vi "Optoelectronic.vi"(0 "Function":T30=enum."Set Parameter Analyzer", 5 "Light Settings":T7={"Laser Settings"={"Wavelength"=enum."365 nm", "Power"=enum."100%"}, "Spectrometer Settings"={"Confocal Hole Size (µm)"=150.0, "Grating"=1, "Detector"=enum."InGaAs Array"}} {"Spectrometer Settings"."Grating" items=["1800 l/mm", "150 l/mm"]}, 7 "Electrical Settings":T14={"SMU1 - Sampling"={"Source"=10.0, "Compliance"=1e-05, "Mode"=0, "Function"=FALSE}, "SMU2 - Sampling"={"Source"=10.0, "Compliance"=1e-05, "Mode"=0, "Function"=FALSE}, "SMU3 - Sampling"={"Source"=10.0, "Compliance"=1e-05, "Mode"=0, "Function"=FALSE}, "SMU4 - Sampling"={"Source"=10.0, "Compliance"=1e-05, "Mode"=0, "Function"=FALSE}} {"SMU4 - Sampling"."Mode" items=["V", "I", "Common"]; "SMU4 - Sampling"."Compliance" format="%^.2e"; "SMU4 - Sampling"."Source" format="%^.3e"; "SMU3 - Sampling"."Mode" items=["V", "I", "Common"]; "SMU3 - Sampling"."Compliance" format="%^.2e"; "SMU3 - Sampling"."Source" format="%^.3e"; "SMU2 - Sampling"."Mode" items=["V", "I", "Common"]; "SMU2 - Sampling"."Compliance" format="%^.2e"; "SMU2 - Sampling"."Source" format="%^.3e"; "SMU1 - Sampling"."Mode" items=["V", "I", "Common"]; "SMU1 - Sampling"."Compliance" format="%^.2e"; "SMU1 - Sampling"."Source" format="%^.3e"}, 9 "Acquisition Settings":T32={"Acquisition Mode"=enum."Single Window", "Spectal Position (nm)"=480.0, "From (nm)"=632.0, "To (nm)"=1000.0, "Integration Time (s)"=3.0, "Number of Accumulations"=3, "AutoScanning"=FALSE, "Spike Removal"=FALSE}, 11 "error in (no error)":errorcluster, 12 "Message Queues":T16, 13 "Notifiers":T17, 14 "Refnums":T1) -> (15 "error out":errorcluster)   [LabVIEW 2014]
uses:
  Hardware Control/Spectrometer/Acquisition Settings.ctl
  Hardware Control/Parameter Analyzer/Parameter Analyzer Sampling Parameters.ctl
  Optoelectronic Funtions.ctl
  support/Notifiers/Notifiers.ctl
  support/Message Handler Loop Notifiers.ctl
  Hardware Control/Parameter Analyzer/Parameter Analyzer Notifiers.ctl
  Hardware Control/Switching Matrix/Switching Matrix Notifiers.ctl
  Hardware Control/Stress Control/StressControl Notifiers.ctl
  Hardware Control/Spectrometer/Spectrometer Notifiers.ctl
  Hardware Control/Switches and Mirrors/SwitchesMirrors Notifiers.ctl
  Hardware Control/Camera/Camera Notifiers.ctl
  Hardware Control/XYZ Stage/XYZ Notifications.ctl
  Hardware Control/Autofocus/Autofocus Notifiers.ctl
  Optoelectronic Notifiers.ctl
  Save Data/SaveData Notifiers.ctl
  Instrument Sequence/Instrument Sequence Notifiers.ctl
  support/Message Queue/All Message Queues.ctl
  support/Message Queue/Message Cluster.ctl
  Optoelectronic Electrical Settings.ctl
  Hardware Control/Parameter Analyzer/Parameter Analyzer SMU Sampling.ctl
  Optoelectronic Light Settings.ctl
  Optoelectronic Laser Settings.ctl
  Hardware Control/Spectrometer/Laser.ctl
  Optoelectronic Power.ctl
  Hardware Control/Spectrometer/Grating Detector Settings.ctl
  Hardware Control/Spectrometer/Grating.ctl
  Hardware Control/Spectrometer/Detector.ctl
  Hardware Control/Parameter Analyzer/Voltage Plot.ctl
  Hardware Control/Parameter Analyzer/Current Plot.ctl
  support/Instrument Status.ctl
  Optoelectronic Refnums.ctl
  Plot Data/Optical Spectrum Plot Refnum.ctl
  Plot Data/Electrical Data Plot Refnums.ctl
  support/Status of All Instruments.ctl
  Hardware Control/Parameter Analyzer/Parameter Analyzer Data.ctl
  Hardware Control/Parameter Analyzer/Parameter Analyzer Config.ctl
  Hardware Control/Parameter Analyzer/Parameter Analyzer Integration Parameters.ctl
  Hardware Control/Parameter Analyzer/Parameter Analyzer SMU Sweeping.ctl
  Hardware Control/Parameter Analyzer/Parameter Analyzer Sweep Spacing.ctl
  Hardware Control/Parameter Analyzer/Parameter Analyzer SMU Range.ctl
  Hardware Control/Parameter Analyzer/Parameter Analyzer Stop Sampling Conditions.ctl
  Hardware Control/Parameter Analyzer/Parameter Analyzer Refnums.ctl
  Hardware Control/Parameter Analyzer/Parameter Analyzer Initialization.ctl
  Hardware Control/Switching Matrix/Switching Matrix Data.ctl
  Hardware Control/Switching Matrix/Switching Matrix Config.ctl
  Hardware Control/Switching Matrix/Switching Matrix Refnums.ctl
  Hardware Control/Switching Matrix/Switching Matrix Initialization.ctl
  Hardware Control/Stress Control/StressControl Data.ctl
  Hardware Control/Stress Control/StressControl Config.ctl
  Hardware Control/Stress Control/StressControl Refnums.ctl
  Hardware Control/Stress Control/StressControl Initialization.ctl
  Hardware Control/Spectrometer/Spectrometer Data.ctl
  Hardware Control/Spectrometer/Spectrometer Config.ctl
  Hardware Control/Spectrometer/Laser Settings.ctl
  Hardware Control/Spectrometer/Filter.ctl
  Hardware Control/Spectrometer/Spectrometer Refnum.ctl
  Hardware Control/Spectrometer/Spectrometer Initialization.ctl
  Hardware Control/Switches and Mirrors/SwitchesMirrors Data.ctl
  Hardware Control/Switches and Mirrors/SwitchesMirrors Config.ctl
  Hardware Control/Switches and Mirrors/SwitchesMirrors Status.ctl
  Hardware Control/Switches and Mirrors/SwitchesMirrors Refnum.ctl
  Hardware Control/Switches and Mirrors/SwitchesMirrors Initialize.ctl
  Hardware Control/Camera/Camera Data.ctl
  Hardware Control/Camera/Camera Config.ctl
  Hardware Control/Camera/Camera Settings.ctl
  Hardware Control/Camera/Camera Refnums.ctl
  Hardware Control/Camera/Camera Initialization.ctl
  Hardware Control/XYZ Stage/XYZ Data.ctl
  Hardware Control/XYZ Stage/XYZ Config.ctl
  Hardware Control/XYZ Stage/XYZ Connection Settings.ctl
  Hardware Control/XYZ Stage/XYZ Stage Control.ctl
  Hardware Control/XYZ Stage/XYZ Coordinate Control.ctl
  Hardware Control/XYZ Stage/XYZ Refnums.ctl
  Hardware Control/XYZ Stage/XYZ Initialization.ctl
  Hardware Control/Autofocus/AutoFocus Data.ctl
  Hardware Control/Autofocus/AutoFocus Config.ctl
  Hardware Control/Autofocus/ZScan.ctl
  <vilib>/Analysis/Matrix/Datatypes/RealMatrix.ctl
  Hardware Control/Autofocus/AutoFocus Refnums.ctl
  Hardware Control/Autofocus/Target Refnums.ctl
  Hardware Control/Autofocus/AutoFocus Initialize.ctl
  Hardware Control/Spectrometer/Spectral Data.ctl
  Hardware Control/Parameter Analyzer/Electrical Data.ctl
  support/Instrument Status State.ctl
  Optoelectronic Measurement.ctl
  support/Message Queue/Message Queue.lvlib
  <vilib>/Analysis/Matrix/NI_Matrix.lvlib
panel:
  out "Instrument Status":T4
  in  "Optical Spectrum":enum32{"Energy", "Wavelength", "Raman Shift"}(tab)
  out "Optical Spectrum vs Energy":cluster{"data":dbl[], "data":dbl[]}(graph)
  out "Optical Spectrum vs Wavelength":cluster{"data":dbl[], "data":dbl[]}(graph)
  out "Optical Spectrum vs Raman Shift":cluster{"data":dbl[], "data":dbl[]}(graph)
  out "Current Plot":T5=[{"Time"=[0.0, 0.30000000000000004, 0.6000000000000001, 0.9, 1.2000000000000002, 1.5, 1.8, 2.1, 2.4000000000000004, 2.7, 3.0, 3.3000000000000003, 3.6, 3.9000000000000004, 4.2, 4.5, 4.800000000000001, 5.1000000000000005, 5.4, 5.7, 6.0, 6.300000000000001, 6.6000000000000005, 6.9, 7.2, 7.5, 7.800000000000001, 8.1, 8.4, 8.700000000000001, 9.0, 9.3, 9.600000000000001, 9.9, 10.200000000000001, 10.5, 10.8, 11.100000000000001, 11.4, 11.700000000000001, 12.0, 12.3, 12.600000000000001, 12.9, 13.200000000000001, 13.5, 13.8, 14.100000000000001, 14.4, 14.700000000000001, 15.0, 15.3, 15.600000000000001, 15.9, 16.2, 16.5, 16.8, 17.1, 17.400000000000002, 17.7], "SMU4"=[9.99995e-06, 9.99995e-06, 9.99995e-06, 9.99997e-06, 9.99997e-06, 9.99997e-06, 9.99997e-06, 9.999980000000001e-06, 9.99997e-06, 9.999980000000001e-06, 9.99997e-06, 9.999980000000001e-06, 9.99997e-06, 9.99997e-06, 9.99997e-06, 9.99996e-06, 9.99996e-06, 9.99996e-06, 9.99996e-06, 9.99997e-06, 9.99997e-06, 9.999980000000001e-06, 9.99997e-06, 9.99997e-06, 9.99997e-06, 9.99997e-06, 9.99997e-06, 9.999980000000001e-06, 9.999980000000001e-06, 9.99996e-06, 9.99997e-06, 9.99996e-06, 9.99997e-06, 9.99997e-06, 9.99997e-06, 9.99997e-06, 9.999980000000001e-06, 9.99997e-06, 9.999980000000001e-06, 9.999980000000001e-06, 9.99997e-06, 9.99997e-06, 9.99997e-06, 9.99996e-06, 9.99996e-06, 9.99997e-06, 9.99997e-06, 9.99996e-06, 9.99996e-06, 9.99997e-06, 9.99997e-06, 9.99997e-06, 9.99997e-06, 9.99997e-06, 9.99996e-06, 9.99997e-06, 9.99997e-06, 9.99997e-06, 9.99997e-06, 9.99996e-06]}, {"Time"=[0.0, 0.30000000000000004, 0.6000000000000001, 0.9, 1.2000000000000002, 1.5, 1.8, 2.1, 2.4000000000000004, 2.7, 3.0, 3.3000000000000003, 3.6, 3.9000000000000004, 4.2, 4.5, 4.800000000000001, 5.1000000000000005, 5.4, 5.7, 6.0, 6.300000000000001, 6.6000000000000005, 6.9, 7.2, 7.5, 7.800000000000001, 8.1, 8.4, 8.700000000000001, 9.0, 9.3, 9.600000000000001, 9.9, 10.200000000000001, 10.5, 10.8, 11.100000000000001, 11.4, 11.700000000000001, 12.0, 12.3, 12.600000000000001, 12.9, 13.200000000000001, 13.5, 13.8, 14.100000000000001, 14.4, 14.700000000000001, 15.0, 15.3, 15.600000000000001, 15.9, 16.2, 16.5, 16.8, 17.1, 17.400000000000002, 17.7], "SMU4"=[-1.00004e-05, -1.000039e-05, -1.000039e-05, -1.0000409999999999e-05, -1.000039e-05, -1.000039e-05, -1.00004e-05, -1.000043e-05, -1.000042e-05, -1.0000409999999999e-05, -1.000039e-05, -1.000039e-05, -1.0000409999999999e-05, -1.00004e-05, -1.000038e-05, -1.000038e-05, -1.000039e-05, -1.000037e-05, -1.000038e-05, -1.000039e-05, -1.000039e-05, -1.000039e-05, -1.000039e-05, -1.000039e-05, -1.00004e-05, -1.000037e-05, -1.000038e-05, -1.000039e-05, -1.00004e-05, -1.00004e-05, -1.00004e-05, -1.000037e-05, -1.000037e-05, -1.000037e-05, -1.000036e-05, -1.000039e-05, -1.000038e-05, -1.000037e-05, -1.000036e-05, -1.000037e-05, -1.000038e-05, -1.000037e-05, -1.000038e-05, -1.000036e-05, -1.000037e-05, -1.000037e-05, -1.000037e-05, -1.000039e-05, -1.000038e-05, -1.000036e-05, -1.000037e-05, -1.000039e-05, -1.000036e-05, -1.000037e-05, -1.000038e-05, -1.00004e-05, -1.0000409999999999e-05, -1.000038e-05, -1.000038e-05, -1.00004e-05]}]
  out "Voltage Plot":T6=[{"Time"=[0.0, 0.30000000000000004, 0.6000000000000001, 0.9, 1.2000000000000002, 1.5, 1.8, 2.1, 2.4000000000000004, 2.7, 3.0, 3.3000000000000003, 3.6, 3.9000000000000004, 4.2, 4.5, 4.800000000000001, 5.1000000000000005, 5.4, 5.7, 6.0, 6.300000000000001, 6.6000000000000005, 6.9, 7.2, 7.5, 7.800000000000001, 8.1, 8.4, 8.700000000000001, 9.0, 9.3, 9.600000000000001, 9.9, 10.200000000000001, 10.5, 10.8, 11.100000000000001, 11.4, 11.700000000000001, 12.0, 12.3, 12.600000000000001, 12.9, 13.200000000000001, 13.5, 13.8, 14.100000000000001, 14.4, 14.700000000000001, 15.0, 15.3, 15.600000000000001, 15.9, 16.2, 16.5, 16.8, 17.1, 17.400000000000002, 17.7], "SMU4"=[9.99995e-06, 9.99995e-06, 9.99995e-06, 9.99997e-06, 9.99997e-06, 9.99997e-06, 9.99997e-06, 9.999980000000001e-06, 9.99997e-06, 9.999980000000001e-06, 9.99997e-06, 9.999980000000001e-06, 9.99997e-06, 9.99997e-06, 9.99997e-06, 9.99996e-06, 9.99996e-06, 9.99996e-06, 9.99996e-06, 9.99997e-06, 9.99997e-06, 9.999980000000001e-06, 9.99997e-06, 9.99997e-06, 9.99997e-06, 9.99997e-06, 9.99997e-06, 9.999980000000001e-06, 9.999980000000001e-06, 9.99996e-06, 9.99997e-06, 9.99996e-06, 9.99997e-06, 9.99997e-06, 9.99997e-06, 9.99997e-06, 9.999980000000001e-06, 9.99997e-06, 9.999980000000001e-06, 9.999980000000001e-06, 9.99997e-06, 9.99997e-06, 9.99997e-06, 9.99996e-06, 9.99996e-06, 9.99997e-06, 9.99997e-06, 9.99996e-06, 9.99996e-06, 9.99997e-06, 9.99997e-06, 9.99997e-06, 9.99997e-06, 9.99997e-06, 9.99996e-06, 9.99997e-06, 9.99997e-06, 9.99997e-06, 9.99997e-06, 9.99996e-06]}, {"Time"=[0.0, 0.30000000000000004, 0.6000000000000001, 0.9, 1.2000000000000002, 1.5, 1.8, 2.1, 2.4000000000000004, 2.7, 3.0, 3.3000000000000003, 3.6, 3.9000000000000004, 4.2, 4.5, 4.800000000000001, 5.1000000000000005, 5.4, 5.7, 6.0, 6.300000000000001, 6.6000000000000005, 6.9, 7.2, 7.5, 7.800000000000001, 8.1, 8.4, 8.700000000000001, 9.0, 9.3, 9.600000000000001, 9.9, 10.200000000000001, 10.5, 10.8, 11.100000000000001, 11.4, 11.700000000000001, 12.0, 12.3, 12.600000000000001, 12.9, 13.200000000000001, 13.5, 13.8, 14.100000000000001, 14.4, 14.700000000000001, 15.0, 15.3, 15.600000000000001, 15.9, 16.2, 16.5, 16.8, 17.1, 17.400000000000002, 17.7], "SMU4"=[-1.00004e-05, -1.000039e-05, -1.000039e-05, -1.0000409999999999e-05, -1.000039e-05, -1.000039e-05, -1.00004e-05, -1.000043e-05, -1.000042e-05, -1.0000409999999999e-05, -1.000039e-05, -1.000039e-05, -1.0000409999999999e-05, -1.00004e-05, -1.000038e-05, -1.000038e-05, -1.000039e-05, -1.000037e-05, -1.000038e-05, -1.000039e-05, -1.000039e-05, -1.000039e-05, -1.000039e-05, -1.000039e-05, -1.00004e-05, -1.000037e-05, -1.000038e-05, -1.000039e-05, -1.00004e-05, -1.00004e-05, -1.00004e-05, -1.000037e-05, -1.000037e-05, -1.000037e-05, -1.000036e-05, -1.000039e-05, -1.000038e-05, -1.000037e-05, -1.000036e-05, -1.000037e-05, -1.000038e-05, -1.000037e-05, -1.000038e-05, -1.000036e-05, -1.000037e-05, -1.000037e-05, -1.000037e-05, -1.000039e-05, -1.000038e-05, -1.000036e-05, -1.000037e-05, -1.000039e-05, -1.000036e-05, -1.000037e-05, -1.000038e-05, -1.00004e-05, -1.0000409999999999e-05, -1.000038e-05, -1.000038e-05, -1.00004e-05]}]
  in  "Sampling Parameters":T31={"Initial Interval (s)"=0.1, "Number of Samples"=60, "Total Sampling Time (s)"=10.0, "Hold Time (s)"=0.0, "Sampling Mode"=0, "Sampling Time"=0} {"Sampling Time" items=["Auto (linear only)", "No Limit", "Set Limit"]; "Sampling Mode" items=["Linear", "Log10", "Log25", "Log50", "Thinned Out"]; "Hold Time (s)" format="%.4f"; "Total Sampling Time (s)" format="%.1f"; "Initial Interval (s)" format="%^.3e"}
  # "LICENSED MATERIALS – PROPERTY OF IBM\nCopyright IBM Corp. 2016,\nALL RIGHTS RESERVED"
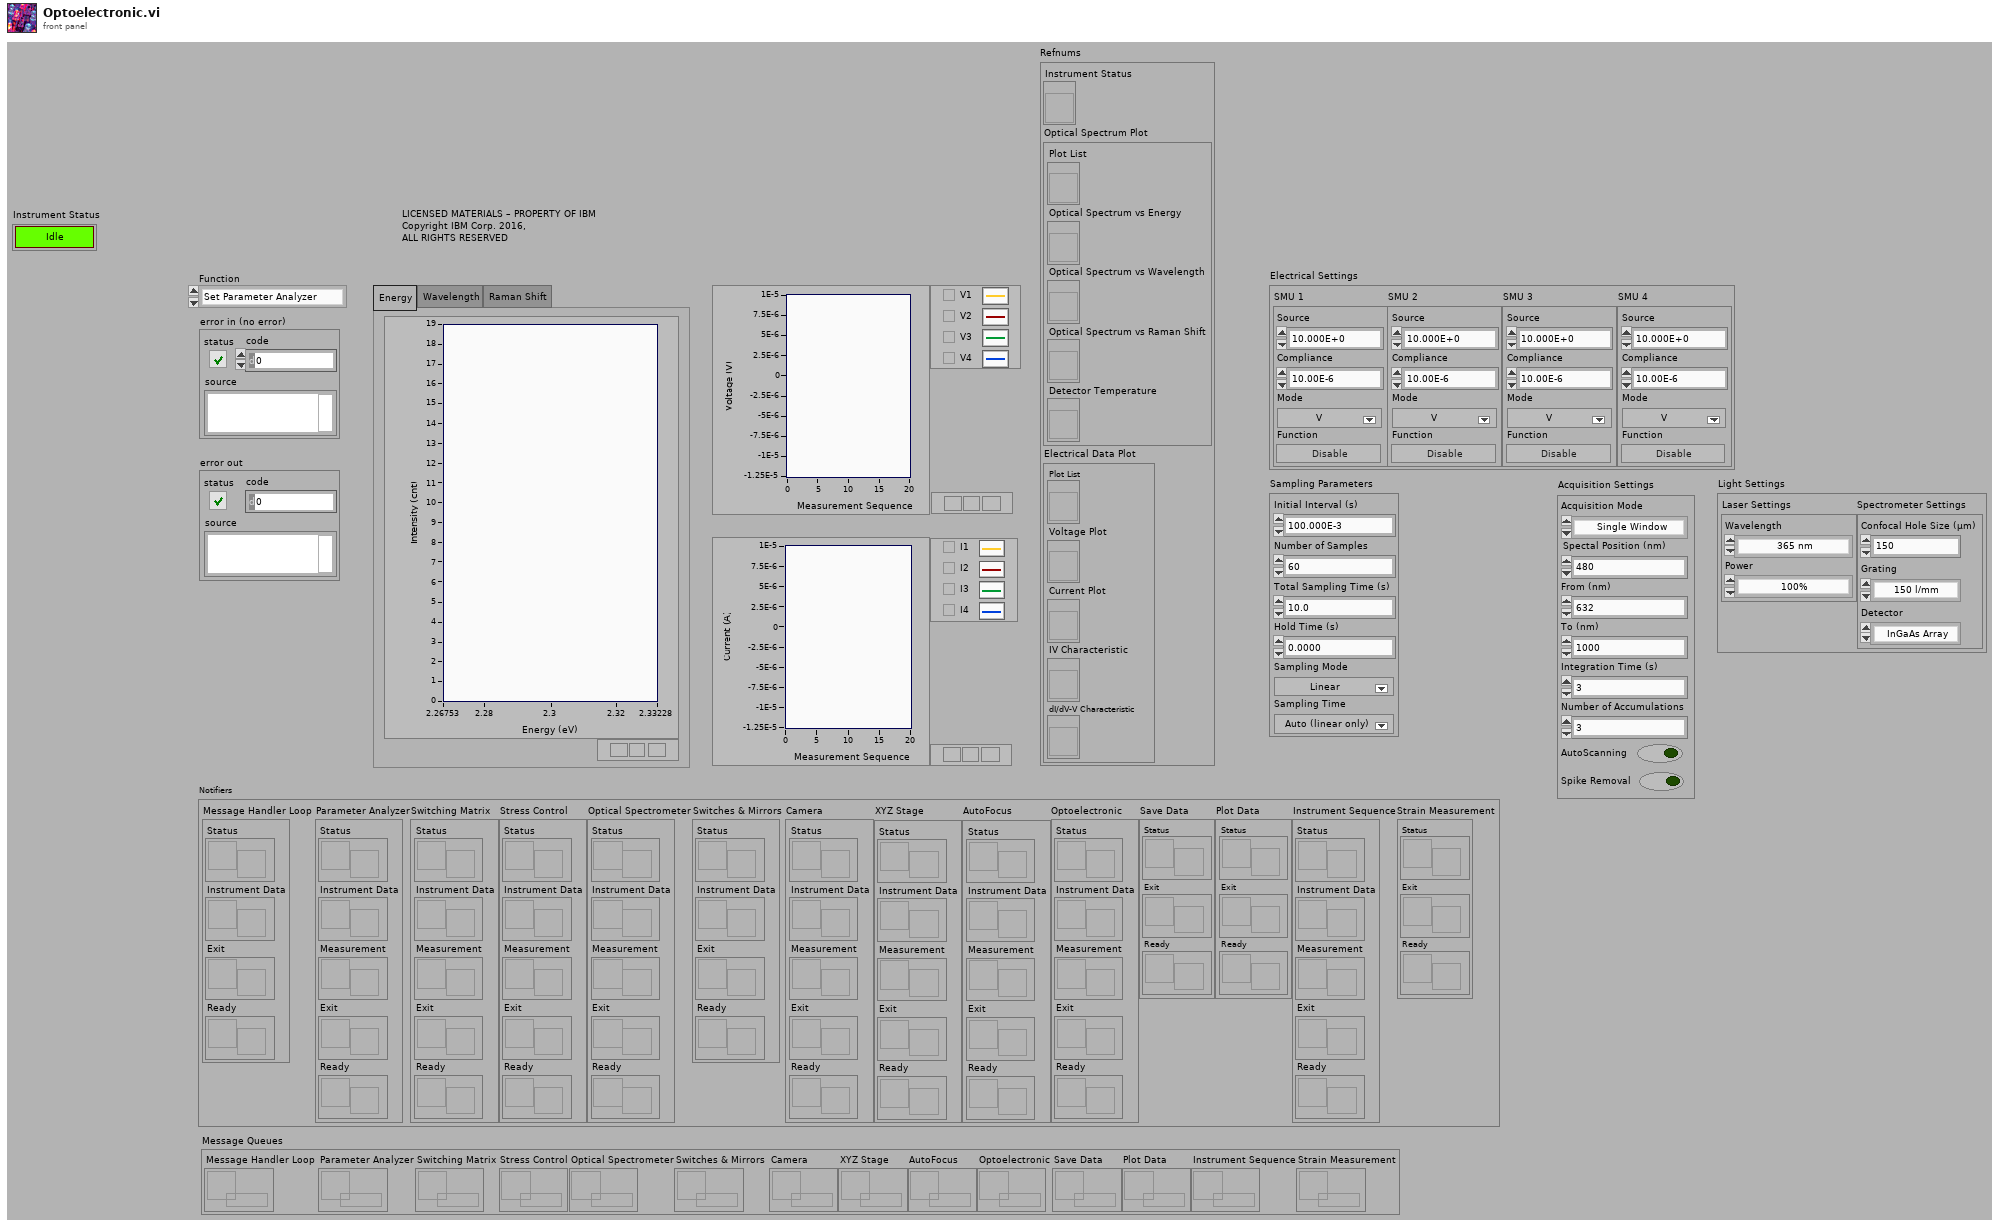
[diagram p1: front panel]
types:
  T1 = typedef "Optoelectronic Refnums.ctl" = cluster{"Instrument Status":refnum<vi>, "Optical Spectrum Plot":T2, "Electrical Data Plot":T3}
  T2 = typedef "Optical Spectrum Plot Refnum.ctl" = cluster{"Plot List":refnum<vi>, "Optical Spectrum vs Energy":refnum<vi>, "Optical Spectrum vs Wavelength":refnum<vi>, "Optical Spectrum vs Raman Shift":refnum<vi>, "Detector Temperature":refnum<vi>}
  T3 = typedef "Electrical Data Plot Refnums.ctl" = cluster{"Plot List":refnum<vi>, "Voltage Plot":refnum<vi>, "Current Plot":refnum<vi>, "IV Characteristic":refnum<vi>, "dI/dV-V Characteristic":refnum<vi>}
  T4 = typedef "Instrument Status.ctl" = bool
  T5 = typedef "Current Plot.ctl" = cluster{"Time":dbl[], "SMU4":dbl[]}[]
  T6 = typedef "Voltage Plot.ctl" = cluster{"Time":dbl[], "SMU4":dbl[]}[]
  T7 = typedef "Optoelectronic Light Settings.ctl" = cluster{"Laser Settings":T8, "Spectrometer Settings":T11}
  T8 = typedef "Optoelectronic Laser Settings.ctl" = cluster{"Wavelength":T9, "Power":T10}
  T9 = typedef "Laser.ctl" = enum16{"633 nm", "784 nm", "532 nm", "365 nm"}
  T10 = typedef "Optoelectronic Power.ctl" = enum16{"100%", "50%", "25%", "10%", "1%", "0.1%", "0.01%", "OFF"}
  T11 = typedef "Grating Detector Settings.ctl" = cluster{"Confocal Hole Size (µm)":dbl, "Grating":T12, "Detector":T13}
  T12 = typedef "Grating.ctl" = u16
  T13 = typedef "Detector.ctl" = enum16{"InGaAs Array", "Silicon CCD"}
  T14 = typedef "Optoelectronic Electrical Settings.ctl" = cluster{"SMU1 - Sampling":T15, "SMU2 - Sampling":T15, "SMU3 - Sampling":T15, "SMU4 - Sampling":T15}
  T15 = typedef "Parameter Analyzer SMU Sampling.ctl" = cluster{"Source":dbl, "Compliance":dbl, "Mode":u32, "Function":bool}
  T16 = typedef "Message Queue.lvlib/All Message Queues.ctl" = cluster{"Message Handler Loop":refnum<queue>, "Parameter Analyzer":refnum<queue>, "Switching Matrix":refnum<queue>, "Stress Control":refnum<queue>, "Optical Spectrometer":refnum<queue>, "Switches & Mirrors":refnum<queue>, "Camera":refnum<queue>, "XYZ Stage":refnum<queue>, "AutoFocus":refnum<queue>, "Optoelectronic":refnum<queue>, "Save Data":refnum<queue>, "Plot Data":refnum<queue>, "Instrument Sequence":refnum<queue>, "Strain Measurement":refnum<queue>}
  T17 = typedef "Notifiers.ctl" = cluster{"Message Handler Loop":T18, "Parameter Analyzer":T19, "Switching Matrix":T20, "Stress Control":T21, "Optical Spectrometer":T22, "Switches & Mirrors":T23, "Camera":T24, "XYZ Stage":T25, "AutoFocus":T26, "Optoelectronic":T27, "Save Data":T28, "Plot Data":T28, "Instrument Sequence":T29, "Strain Measurement":cluster{"Status":refnum<notifier>, "Exit":refnum<notifier>, "Ready":refnum<notifier>}}
  T18 = typedef "Message Handler Loop Notifiers.ctl" = cluster{"Status":refnum<notifier>, "Instrument Data":refnum<notifier>, "Exit":refnum<notifier>, "Ready":refnum<notifier>}
  T19 = typedef "Parameter Analyzer Notifiers.ctl" = cluster{"Status":refnum<notifier>, "Instrument Data":refnum<notifier>, "Measurement":refnum<notifier>, "Exit":refnum<notifier>, "Ready":refnum<notifier>}
  T20 = typedef "Switching Matrix Notifiers.ctl" = cluster{"Status":refnum<notifier>, "Instrument Data":refnum<notifier>, "Measurement":refnum<notifier>, "Exit":refnum<notifier>, "Ready":refnum<notifier>}
  T21 = typedef "StressControl Notifiers.ctl" = cluster{"Status":refnum<notifier>, "Instrument Data":refnum<notifier>, "Measurement":refnum<notifier>, "Exit":refnum<notifier>, "Ready":refnum<notifier>}
  T22 = typedef "Spectrometer Notifiers.ctl" = cluster{"Status":refnum<notifier>, "Instrument Data":refnum<notifier>, "Measurement":refnum<notifier>, "Exit":refnum<notifier>, "Ready":refnum<notifier>}
  T23 = typedef "SwitchesMirrors Notifiers.ctl" = cluster{"Status":refnum<notifier>, "Instrument Data":refnum<notifier>, "Exit":refnum<notifier>, "Ready":refnum<notifier>}
  T24 = typedef "Camera Notifiers.ctl" = cluster{"Status":refnum<notifier>, "Instrument Data":refnum<notifier>, "Measurement":refnum<notifier>, "Exit":refnum<notifier>, "Ready":refnum<notifier>}
  T25 = typedef "XYZ Notifications.ctl" = cluster{"Status":refnum<notifier>, "Instrument Data":refnum<notifier>, "Measurement":refnum<notifier>, "Exit":refnum<notifier>, "Ready":refnum<notifier>}
  T26 = typedef "Autofocus Notifiers.ctl" = cluster{"Status":refnum<notifier>, "Instrument Data":refnum<notifier>, "Measurement":refnum<notifier>, "Exit":refnum<notifier>, "Ready":refnum<notifier>}
  T27 = typedef "Optoelectronic Notifiers.ctl" = cluster{"Status":refnum<notifier>, "Instrument Data":refnum<notifier>, "Measurement":refnum<notifier>, "Exit":refnum<notifier>, "Ready":refnum<notifier>}
  T28 = typedef "SaveData Notifiers.ctl" = cluster{"Status":refnum<notifier>, "Exit":refnum<notifier>, "Ready":refnum<notifier>}
  T29 = typedef "Instrument Sequence Notifiers.ctl" = cluster{"Status":refnum<notifier>, "Instrument Data":refnum<notifier>, "Measurement":refnum<notifier>, "Exit":refnum<notifier>, "Ready":refnum<notifier>}
  T30 = typedef "Optoelectronic Funtions.ctl" = enum16{"Get Instruments Status", "Measure", "Set Parameter Analyzer", "Set Spectrometer", "Set Acquisition", "Update Refnums"}
  T31 = typedef "Parameter Analyzer Sampling Parameters.ctl" = cluster{"Initial Interval (s)":dbl, "Number of Samples":i32, "Total Sampling Time (s)":dbl, "Hold Time (s)":dbl, "Sampling Mode":i32, "Sampling Time":i32}
  T32 = typedef "Acquisition Settings.ctl" = cluster{"Acquisition Mode":enum16{"Single Window", "Multi-Window"}, "Spectal Position (nm)":dbl, "From (nm)":dbl, "To (nm)":dbl, "Integration Time (s)":dbl, "Number of Accumulations":i32, "AutoScanning":bool, "Spike Removal":bool}
  T33 = enum32{"Current & Voltage Traces", "Four | Two Probe"}
  T34 = typedef "Optoelectronic Measurement.ctl" = cluster{"Optical Spectrum":T35, "Electrical Measurement":T36}
  T35 = typedef "Spectral Data.ctl" = cluster{"Intensity":dbl[], "Wavelength":dbl[], "Energy":dbl[], "Raman Shift":dbl[], "Detector Temperature":dbl}
  T36 = typedef "Electrical Data.ctl" = cluster{"Sequence":dbl[], "V1":dbl[], "V2":dbl[], "V3":dbl[], "V4":dbl[], "I1":dbl[], "I2":dbl[], "I3":dbl[], "I4":dbl[]}
  T37 = typedef "Instrument Status State.ctl" = enum16{"Unknown", "Idle", "Standby", "Configuring", "Measuring", "Moving", "Disconnected"}
  T38 = typedef "Status of All Instruments.ctl" = cluster{"Parameter Analyzer":T39, "Swithing Matrix":T48, "Stress Control":T52, "Optical Spectrometer":T56, "Switches & Mirrors":T62, "Camera":T67, "XYZ Stage":T72, "AutoFocus":T79}
  T39 = typedef "Parameter Analyzer Data.ctl" = cluster{"Configuration":T40, "Refnums":T46, "Initialization":T47}
  T40 = typedef "Parameter Analyzer Config.ctl" = cluster{"Parameter Analyzer VISA Session":refnum<visa-resource-name>, "Sweeping Time Parameters":T41, "Acquisition Mode":enum32{"Sweeping Mode", "Sampling Mode"}, "Status Polling Time (ms)":u32, "Comment":string, "SMU 1 - Sweeping":T42, "SMU 2 - Sweeping":T42, "SMU 3 - Sweeping":T42, "SMU 4 - Sweeping":T42, "Sweep Spacing":T43, "Range":T44, "SMU1 - Sampling":T15, "SMU2 - Sampling":T15, "SMU3 - Sampling":T15, "SMU4 - Sampling":T15, "Sampling Time Parameters":T31, "Stop Condition":T45}
  T41 = typedef "Parameter Analyzer Integration Parameters.ctl" = cluster{"Integration Time":u32, "Short Integration Time (s)":dbl, "Long Integration Time (s)":dbl, "Wait Time Parameter":dbl}
  T42 = typedef "Parameter Analyzer SMU Sweeping.ctl" = cluster{"Start / Offset":dbl, "Stop / Ratio":dbl, "Step \n(linear only)":dbl, "Compliance":dbl, "Power \nCompliance":dbl, "Mode":u32, "Function":i32, "Sweep Mode":bool}
  T43 = typedef "Parameter Analyzer Sweep Spacing.ctl" = u16
  T44 = typedef "Parameter Analyzer SMU Range.ctl" = u16
  T45 = typedef "Parameter Analyzer Stop Sampling Conditions.ctl" = cluster{"Enable Delay (s)":dbl, "Name":string, "Threshold":dbl, "num. of events":i32, "Event":i32, "Stop Condition Enable":bool}
  T46 = typedef "Parameter Analyzer Refnums.ctl" = cluster{"Status":refnum<vi>, "Electrical Measurement":refnum<vi>, "Plots":T3, "HP Integration Time":refnum<vi>, "VISA":refnum<vi>, "Sweeping Time Parameters":refnum<vi>, "Acquisition Mode":refnum<vi>, "SMU 1 - Sweeping":refnum<vi>, "SMU 2 - Sweeping":refnum<vi>, "SMU 3 - Sweeping":refnum<vi>, "SMU 4 - Sweeping":refnum<vi>, "Sweep Spacing":refnum<vi>, "Range":refnum<vi>, "SMU1 - Sampling":refnum<vi>, "SMU2 - Sampling":refnum<vi>, "SMU3 - Sampling":refnum<vi>, "SMU4 - Sampling":refnum<vi>, "Sampling Time Parameters":refnum<vi>, "Stop Condition":refnum<vi>, "Instrument Status":refnum<vi>}
  T47 = typedef "Parameter Analyzer Initialization.ctl" = cluster{"Update Visa Session":bool, "Configure Integration Time":bool, "Configure Acquisition Mode":bool, "Update Refnums":bool}
  T48 = typedef "Switching Matrix Data.ctl" = cluster{"Configuration":T49, "Refnums":T50, "Initialization":T51}
  T49 = typedef "Switching Matrix Config.ctl" = cluster{"Switching Matrix VISA Session":refnum<visa-resource-name>, "Connections":cluster{"Connections":bool[], "Connection Type":enum16{"Disconnected", "Make - Break", "Break - Make"}}[]}
  T50 = typedef "Switching Matrix Refnums.ctl" = cluster{"Connections":refnum<vi>, "Instrument Status":refnum<vi>}
  T51 = typedef "Switching Matrix Initialization.ctl" = cluster{"Update Visa Session":bool, "Update Refnums":bool}
  T52 = typedef "StressControl Data.ctl" = cluster{"Configuration":T53, "Refnums":T54, "Initialization":T55}
  T53 = typedef "StressControl Config.ctl" = cluster{"Stress Control VISA Session":refnum<visa-resource-name>, "Axis":i32, "Motion":u16, "Destination (°)":dbl, "Speed (°/s)":dbl, "Position (°)":dbl}
  T54 = typedef "StressControl Refnums.ctl" = cluster{"Instrument Status":refnum<vi>, "Position":refnum<vi>, "Mecahnism Motion":refnum<vi>, "Destination":refnum<vi>, "Apply Stress":refnum<vi>, "Stop":refnum<vi>, "Stress Control VISA":refnum<vi>}
  T55 = typedef "StressControl Initialization.ctl" = cluster{"Update Visa Session":bool, "Update Configuration":bool, "Update Refnums":bool, "Get Position":bool}
  T56 = typedef "Spectrometer Data.ctl" = cluster{"Configuration":T57, "Refnums":T60, "Initialization":T61}
  T57 = typedef "Spectrometer Config.ctl" = cluster{"Laser Settings":T58, "Spectrometer Settings":T11, "Acquisition Settings":T32, "Path":path}
  T58 = typedef "Laser Settings.ctl" = cluster{"Laser Wavelength":T9, "Neutral Density Filter":T59}
  T59 = typedef "Filter.ctl" = enum16{"100%", "50%", "25%", "10%", "1%", "0.1%", "0.01%"}
  T60 = typedef "Spectrometer Refnum.ctl" = cluster{"Instrument Status":refnum<vi>, "Optical Spectrum Plot":T2, "Laser":refnum<vi>, "Filter":refnum<vi>, "Laser ON?":refnum<vi>, "Hole":refnum<vi>, "Grating":refnum<vi>, "Detector":refnum<vi>, "Acquisition Mode":refnum<vi>, "Spectal Position":refnum<vi>, "From":refnum<vi>, "To":refnum<vi>, "Integration Time":refnum<vi>, "Accumulations":refnum<vi>, "AutoScanning":refnum<vi>, "Spike Removal":refnum<vi>, "Acquisition Mode Panel":refnum<vi>}
  T61 = typedef "Spectrometer Initialization.ctl" = cluster{"Connect":bool, "Update Refnums":bool, "Get Configuration":bool}
  T62 = typedef "SwitchesMirrors Data.ctl" = cluster{"Configuration":T63, "Refnums":T65, "Initialize":T66}
  T63 = typedef "SwitchesMirrors Config.ctl" = cluster{"Relay VISA Session":refnum<visa-resource-name>, "Switches":T64, "Delays (ms)":cluster{"Laser":u32, "Video":u32}}
  T64 = typedef "SwitchesMirrors Status.ctl" = cluster{"Laser":bool, "Video":bool}
  T65 = typedef "SwitchesMirrors Refnum.ctl" = cluster{"Instrument Status":refnum<vi>, "Laser":refnum<vi>, "Video":refnum<vi>, "Relay VISA":refnum<vi>}
  T66 = typedef "SwitchesMirrors Initialize.ctl" = cluster{"Update Refnums":bool, "Connect":bool, "Set Configuration":bool}
  T67 = typedef "Camera Data.ctl" = cluster{"Configuration":T68, "Refnums":T70, "Initialization":T71}
  T68 = typedef "Camera Config.ctl" = cluster{"Settings":T69}
  T69 = typedef "Camera Settings.ctl" = cluster{"Pixel clock":i32, "Frame rate":dbl, "Exposure time":dbl, "Master Gain":i32, "Red Gain":i32, "Green Gain":i32, "Blue Gain":i32, "Auto Gain":bool, "White-balance":bool, "Color Correction":bool}
  T70 = typedef "Camera Refnums.ctl" = cluster{"Pixel Clock":refnum<vi>, "Frame Rate":refnum<vi>, "Exposure Time":refnum<vi>, "Master Gain":refnum<vi>, "Red Gain":refnum<vi>, "Green Gain":refnum<vi>, "Blue Gain":refnum<vi>, "Auto Gain":refnum<vi>, "Auto White-balance":refnum<vi>, "Color Correction":refnum<vi>, "Image":refnum<vi>, "Video Button":refnum<vi>, "Instrument Status":refnum<vi>}
  T71 = typedef "Camera Initialization.ctl" = cluster{"Connect":bool, "Update Refnums":bool, "Acquiring?":bool}
  T72 = typedef "XYZ Data.ctl" = cluster{"Configuration":T73, "Refnums":T77, "Initialization":T78}
  T73 = typedef "XYZ Config.ctl" = cluster{"Connection Settings":T74, "Manual Control":T75, "Coordinate Control":T76}
  T74 = typedef "XYZ Connection Settings.ctl" = cluster{"Tango VISA":refnum<visa-resource-name>, "Baudrate":i32, "Show Protocol?":bool}
  T75 = typedef "XYZ Stage Control.ctl" = cluster{"North":bool, "South":bool, "West":bool, "East":bool, "Up":bool, "Down":bool, "Stop":bool, "XY Step":dbl, "Z step":dbl}
  T76 = typedef "XYZ Coordinate Control.ctl" = cluster{"Motion Mode":enum16{"Absolute", "Relative"}, "Destination [mm]":dbl[]}
  T77 = typedef "XYZ Refnums.ctl" = cluster{"Instrument Status":refnum<vi>, "Position":refnum<vi>, "Manual Control":refnum<vi>, "Up":refnum<vi>, "Down":refnum<vi>, "North":refnum<vi>, "South":refnum<vi>, "East":refnum<vi>, "West":refnum<vi>, "Stop":refnum<vi>, "Limits":refnum<vi>}
  T78 = typedef "XYZ Initialization.ctl" = cluster{"Update Visa Session":bool, "Set To Default":bool, "Get Status":bool, "Update Refnums":bool}
  T79 = typedef "AutoFocus Data.ctl" = cluster{"Configuration":T80, "Refnums":T83, "Initialize":T85}
  T80 = typedef "AutoFocus Config.ctl" = cluster{"Matching Criteria":cluster{"Minimum Score":sgl, "Color Score Weight":sgl, "Minimum Contrast":i32, "Match Mode":u32, "Match Feature Mode":u32, "Subpixel Accuracy":bool, "Color Sensitivity":u32, "Search Strategy":u32}, "Z Scan Parameters":T81, "Displacement":dbl, "Transformation Matrix":T82}
  T81 = typedef "ZScan.ctl" = cluster{"Z Range":ext, "Resolution":dbl, "Initial Direction":enum16{"Up", "Down"}, "Focus Threshold":dbl, "Ascent Constant":dbl}
  T82 = typedef "NI_Matrix.lvlib/RealMatrix.ctl" = dbl[][]
  T83 = typedef "AutoFocus Refnums.ctl" = cluster{"Instrument Status":refnum<vi>, "Matching Criteria":refnum<vi>, "Z Scan Parameters":refnum<vi>, "Distance":refnum<vi>, "Transformation Matrix":refnum<vi>, "Match and Edge":T84, "Matching Curves":refnum<vi>, "Tracking":refnum<vi>, "Focus":refnum<vi>, "Find Focus":refnum<vi>, "Set Target":refnum<vi>, "Link Stage & Camera":refnum<vi>, "Align":refnum<vi>}
  T84 = typedef "Target Refnums.ctl" = cluster{"Image":refnum<vi>, "Target":refnum<vi>, "Edge":refnum<vi>, "Target Data":refnum<vi>}
  T85 = typedef "AutoFocus Initialize.ctl" = cluster{"Update Refnums":bool, "Allocate Image Memory":bool, "Set Match Criteria":bool, "Link Stage & Camera":bool, "Set Target":bool, "Find Target":bool}
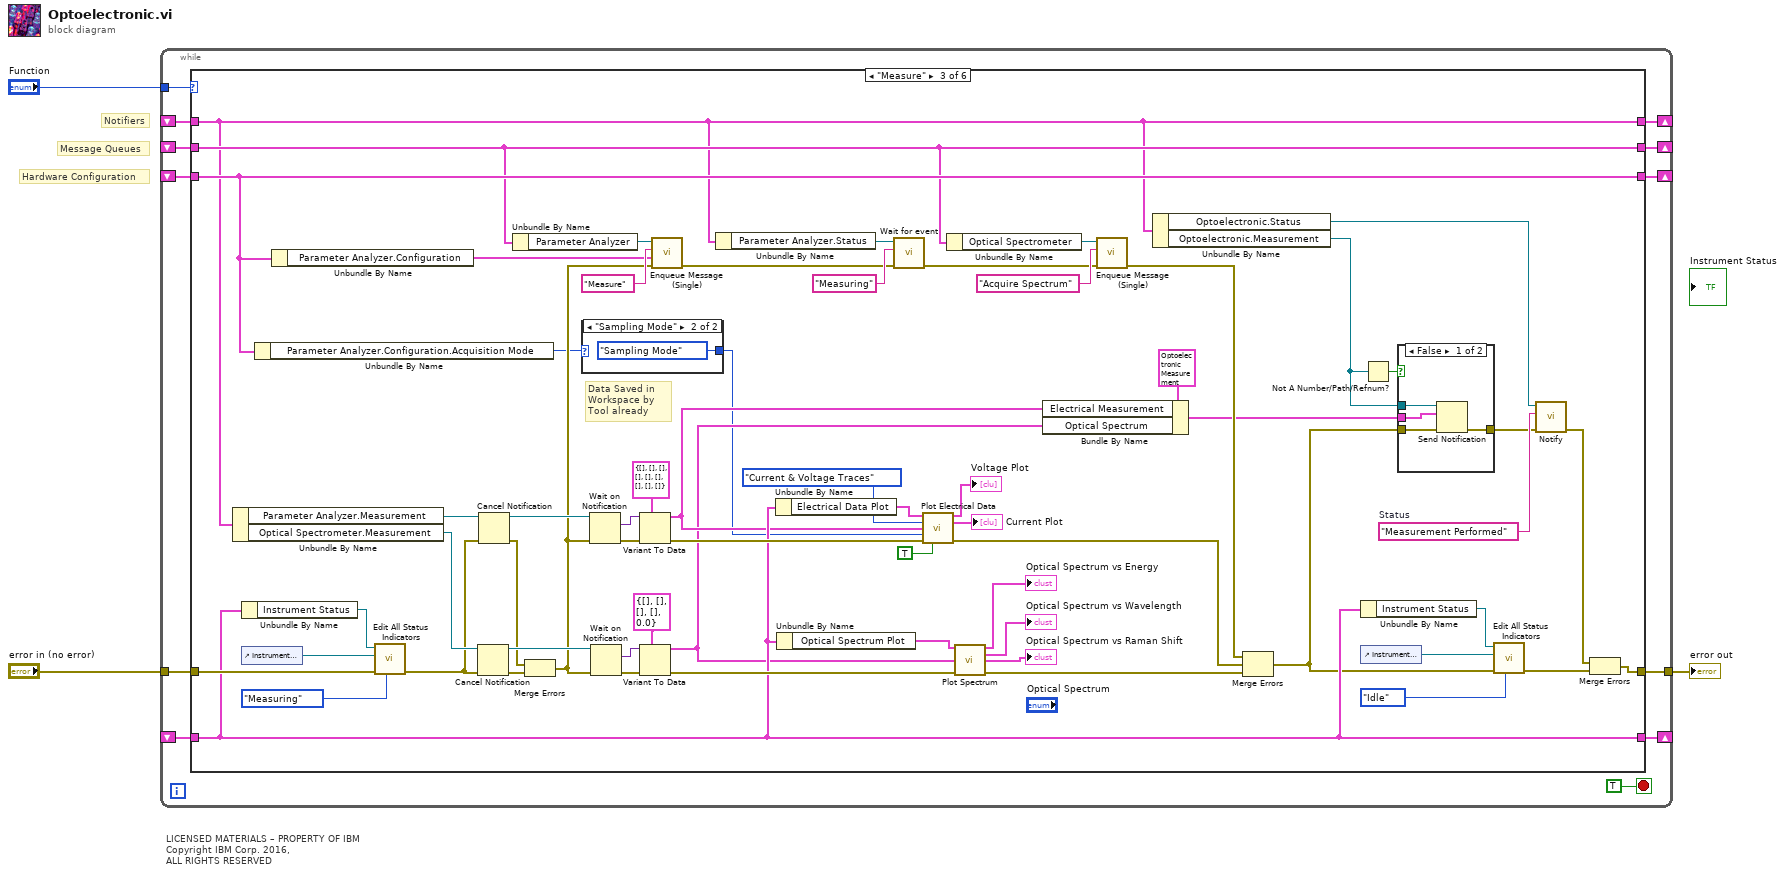
[diagram p0: block diagram]
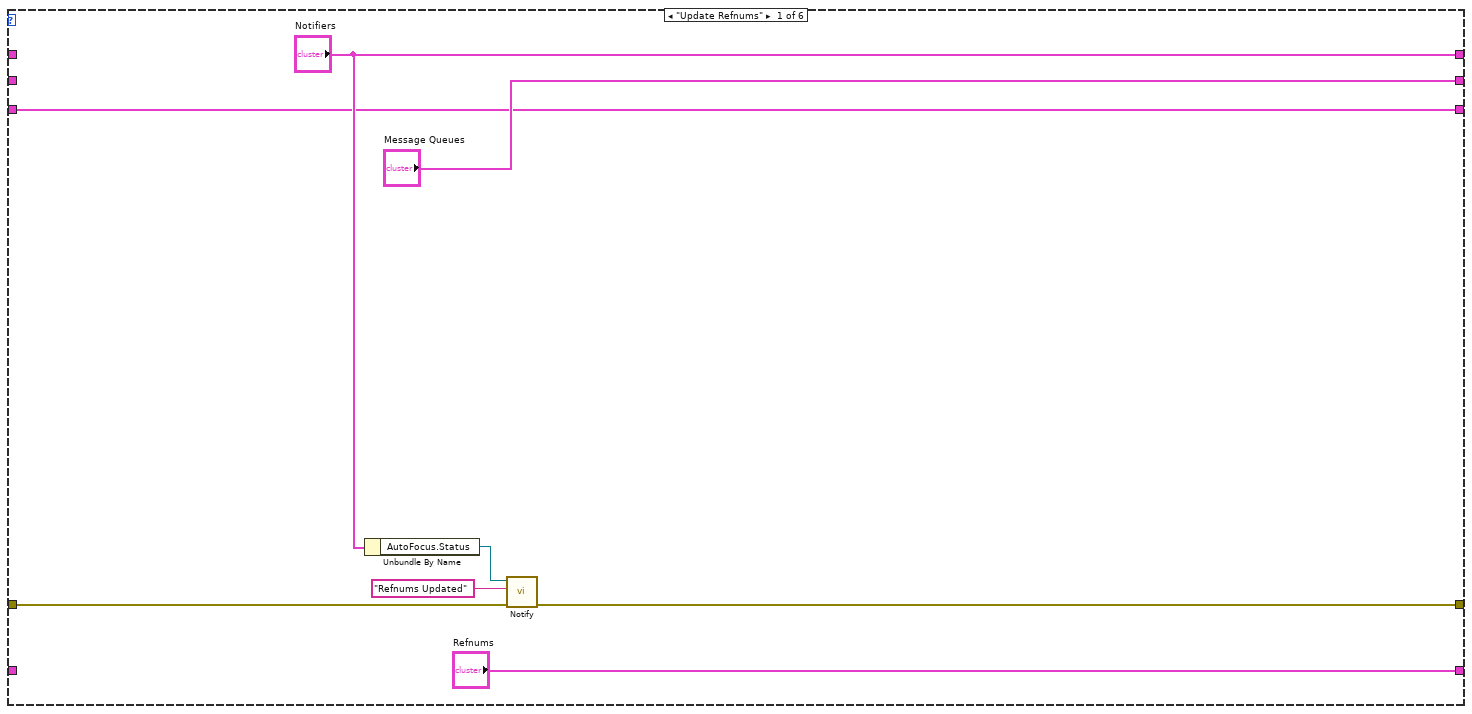
[diagram p2: hidden frame]
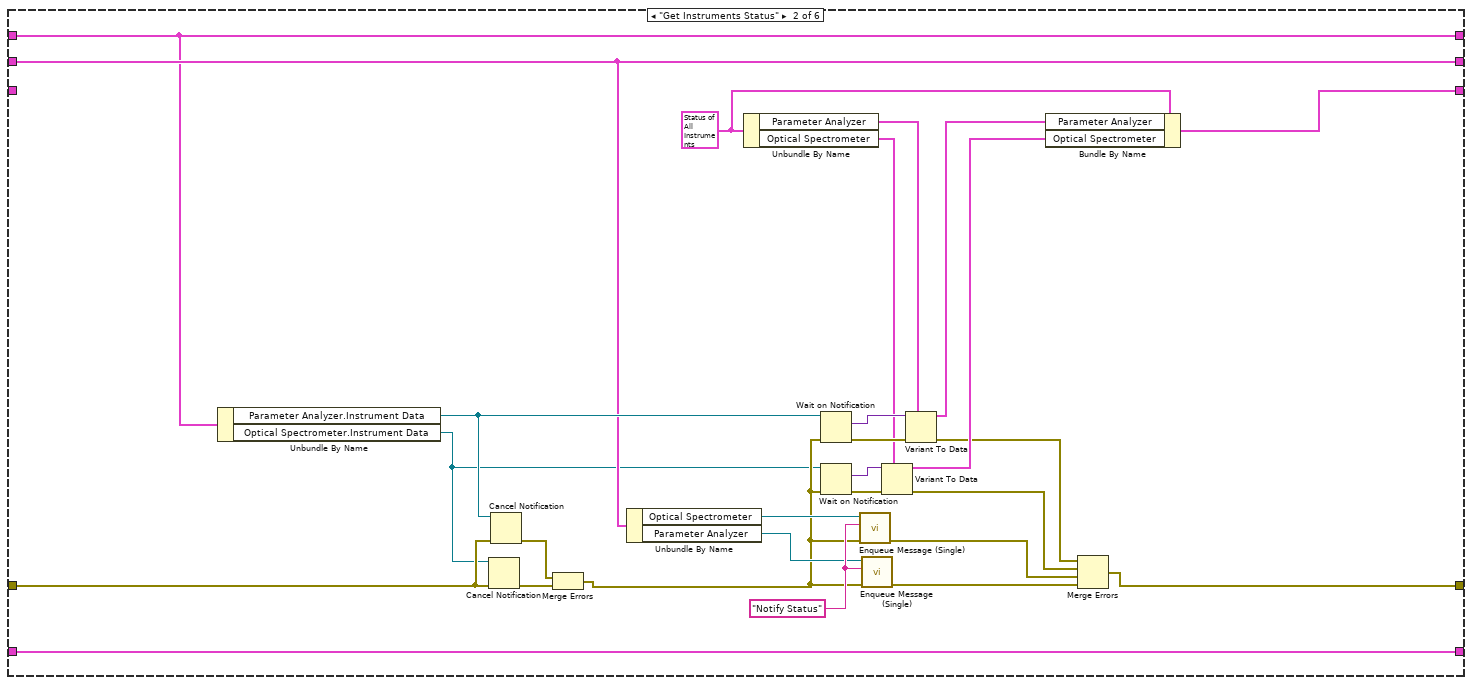
[diagram p3: hidden frame]
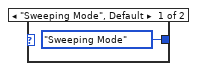
[diagram p4: hidden frame]
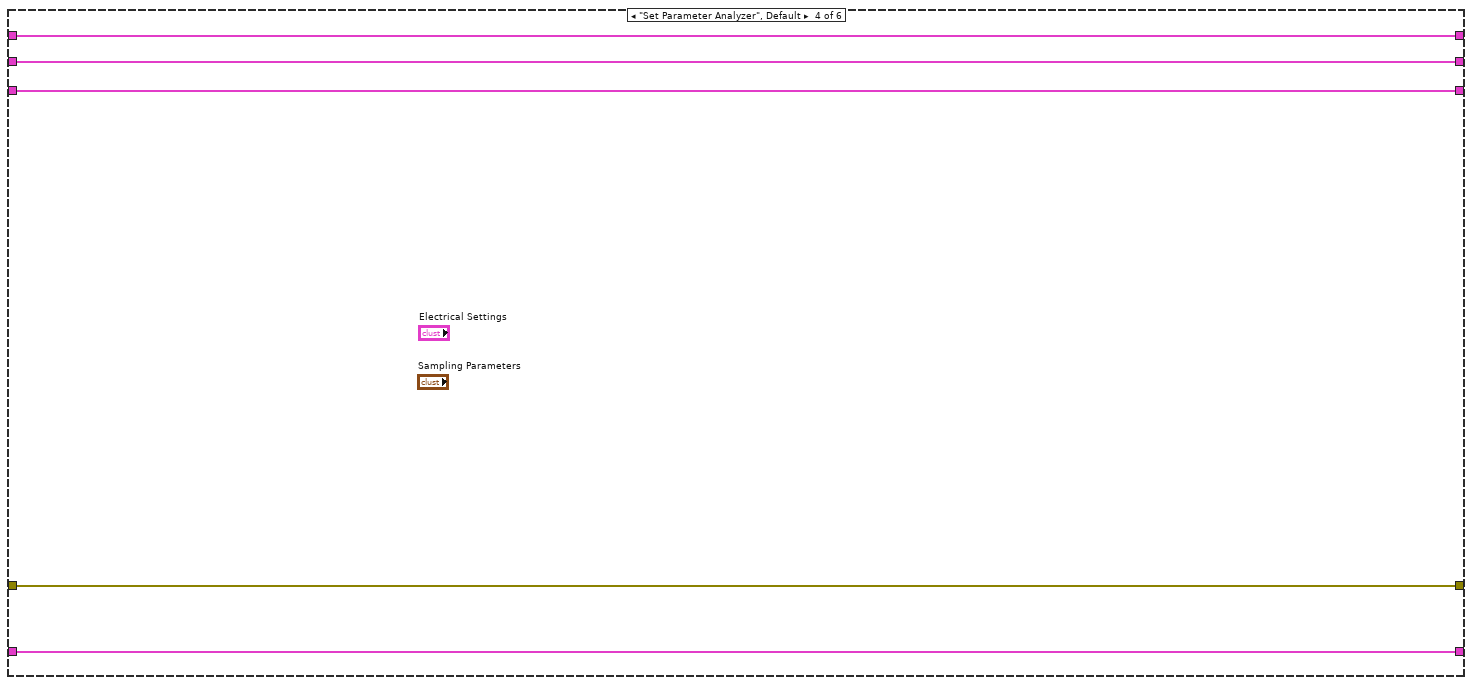
[diagram p6: hidden frame]
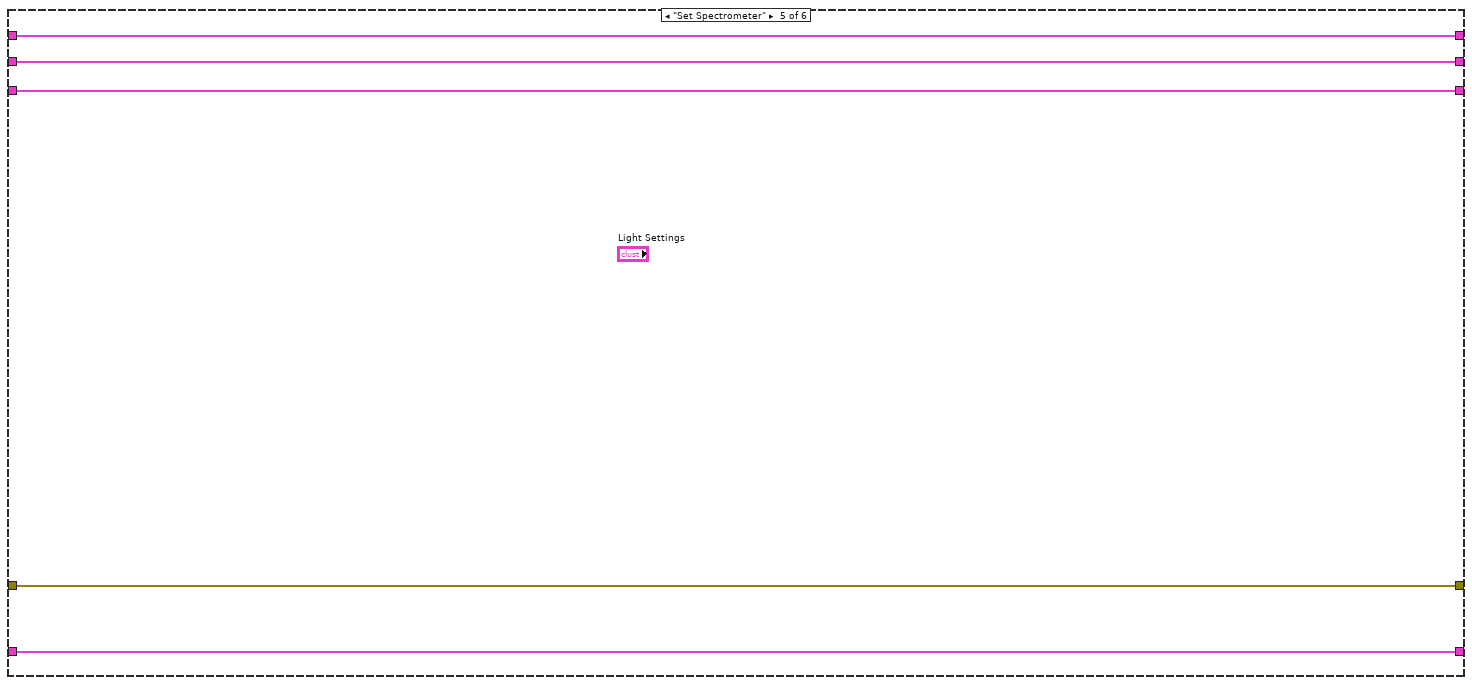
[diagram p7: hidden frame]
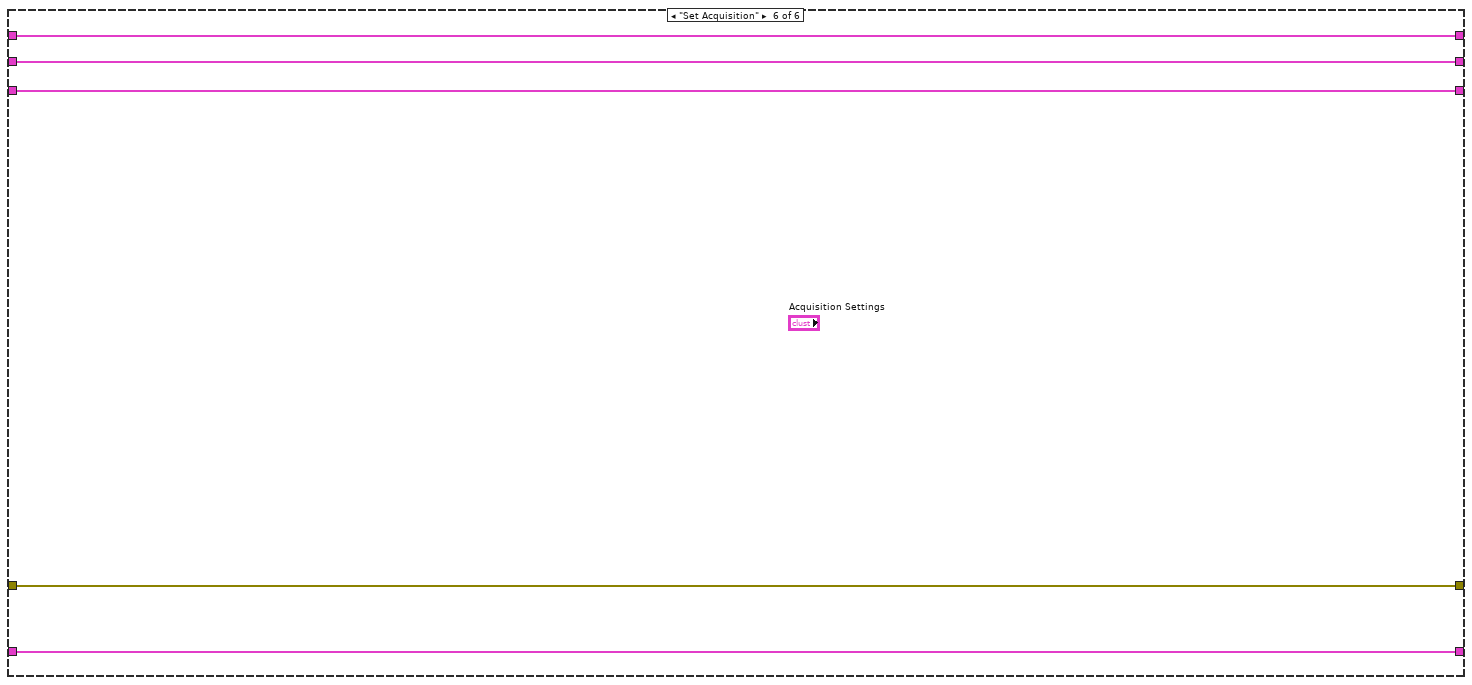
[diagram p8: hidden frame]
diagram:
  # "LICENSED MATERIALS – PROPERTY OF IBM\nCopyright IBM Corp. 2016,\nALL RIGHTS RESERVED"
  # "Hardware Configuration"
  # "Message Queues"
  # "Notifiers"
  n1 = while {
    tunnel: "Function" -> [w14]
    shift-right: [w13] -> _
    shift-left: _ -> [w12]
    shift-right: [w11] -> _
    shift-left: _ -> [w10]
    tunnel: [w9] -> w1
    tunnel: "error in (no error)" -> [w8]
    shift-right: [w5] -> _
    shift-left: _ -> [w4]
    shift-right: [w7] -> _
    shift-left: _ -> [w6]
    stop <- TRUE stop-if-true
    n2 = case shown="\"Measure\"" w14 {
      tunnel: ["Message Queues" w33 w60 w125 w130 w135] -> w13
      tunnel: w12 -> [_ w33 w60 w125 w130 w135]
      tunnel: ["Notifiers" w32 w55 w124 w129 w134] -> w11
      tunnel: w10 -> [_ w32 w55 w124 w129 w134]
      tunnel: [w19 w30 w85 w123 w128 w133] -> w9
      tunnel: w8 -> [w18 w35 w74 w123 w128 w133]
      tunnel: [w17 w34 w61 w122 w127 w132] -> w7
      tunnel: w6 -> [w17 _ w61 w122 w127 w132]
      tunnel: ["Refnums" w31 w70 w121 w126 w131] -> w5
      tunnel: w4 -> [_ w31 w70 w121 w126 w131]
      frame "Update Refnums" {
        n3 = Unbundle By Name("Notifiers") -> ("AutoFocus.Status"=w23:refnum<notifier>)
        n4 = call "Notify.vi"("error in (no error)"=w18, "String"="Refnums Updated", "Notifier in"=w23) -> ("error out"=w19:errorcluster)  [unwired: 8 in]
      }
      frame "Get Instruments Status" {
        w49 = "Notify Status" ("Message")
        w50 = T38 {"Parameter Analyzer"={"Configuration"={"Parameter Analyzer VISA Session"="COM1", "Sweeping Time Parameters"={"Integration Time"=0, "Short Integration Time (s)"=1.0, "Long Integration Time (s)"=0.0, "Wait Time Parameter"=1.0}, "Acquisition Mode"=enum."Sweeping Mode", "Status Polling Time (ms)"=1000, "Comment"="Test VI", "SMU 1 - Sweeping"={"Start / Offset"=0.0, "Stop / Ratio"=1.0, "Step \n(linear only)"=0.01, "Compliance"=0.1, "Power \nCompliance"=0.0, "Mode"=0, "Function"=0, "Sweep Mode"=FALSE}, "SMU 2 - Sweeping"={"Start / Offset"=0.0, "Stop / Ratio"=1.0, "Step \n(linear only)"=0.01, "Compliance"=0.1, "Power \nCompliance"=0.0, "Mode"=0, "Function"=0, "Sweep Mode"=FALSE}, "SMU 3 - Sweeping"={"Start / Offset"=0.0, "Stop / Ratio"=1.0, "Step \n(linear only)"=0.01, "Compliance"=0.1, "Power \nCompliance"=0.0, "Mode"=0, "Function"=0, "Sweep Mode"=FALSE}, "SMU 4 - Sweeping"={"Start / Offset"=0.0, "Stop / Ratio"=1.0, "Step \n(linear only)"=0.01, "Compliance"=0.1, "Power \nCompliance"=0.0, "Mode"=0, "Function"=0, "Sweep Mode"=FALSE}, "Sweep Spacing"=0, "Range"=0, "SMU1 - Sampling"={"Source"=10.0, "Compliance"=1e-05, "Mode"=0, "Function"=FALSE}, "SMU2 - Sampling"={"Source"=10.0, "Compliance"=1e-05, "Mode"=0, "Function"=FALSE}, "SMU3 - Sampling"={"Source"=10.0, "Compliance"=1e-05, "Mode"=0, "Function"=FALSE}, "SMU4 - Sampling"={"Source"=0.1, "Compliance"=60.0, "Mode"=10, "Function"=FALSE}, "Sampling Time Parameters"={"Initial Interval (s)"=0.1, "Number of Samples"=60, "Total Sampling Time (s)"=10.0, "Hold Time (s)"=0.0, "Sampling Mode"=0, "Sampling Time"=0}, "Stop Condition"={"Enable Delay (s)"=0.0, "Name"="", "Threshold"=0.0, "num. of events"=1, "Event"=0, "Stop Condition Enable"=FALSE}}, "Refnums"={"Status"=refnum, "Electrical Measurement"=refnum, "Plots"={"Plot List"=refnum, "Voltage Plot"=refnum, "Current Plot"=refnum, "IV Characteristic"=refnum, "dI/dV-V Characteristic"=refnum}, "HP Integration Time"=refnum, "VISA"=refnum, "Sweeping Time Parameters"=refnum, "Acquisition Mode"=refnum, "SMU 1 - Sweeping"=refnum, "SMU 2 - Sweeping"=refnum, "SMU 3 - Sweeping"=refnum, "SMU 4 - Sweeping"=refnum, "Sweep Spacing"=refnum, "Range"=refnum, "SMU1 - Sampling"=refnum, "SMU2 - Sampling"=refnum, "SMU3 - Sampling"=refnum, "SMU4 - Sampling"=refnum, "Sampling Time Parameters"=refnum, "Stop Condition"=refnum, "Instrument Status"=refnum}, "Initialization"={"Update Visa Session"=FALSE, "Configure Integration Time"=FALSE, "Configure Acquisition Mode"=FALSE, "Update Refnums"=FALSE}}, "Swithing Matrix"={"Configuration"={"Switching Matrix VISA Session"="GPIB0::18::INSTR", "Connections"=[{"Connections"=[FALSE, FALSE, FALSE, FALSE, FALSE, FALSE, FALSE, FALSE, FALSE, FALSE, FALSE, FALSE], "Connection Type"=enum."Disconnected"}, {"Connections"=[FALSE, FALSE, FALSE, FALSE, FALSE, FALSE, FALSE, FALSE, FALSE, FALSE, FALSE, FALSE], "Connection Type"=enum."Disconnected"}, {"Connections"=[FALSE, FALSE, FALSE, FALSE, FALSE, FALSE, FALSE, FALSE, FALSE, FALSE, FALSE, FALSE], "Connection Type"=enum."Disconnected"}, {"Connections"=[FALSE, FALSE, FALSE, FALSE, FALSE, FALSE, FALSE, FALSE, FALSE, FALSE, FALSE, FALSE], "Connection Type"=enum."Disconnected"}, {"Connections"=[FALSE, FALSE, FALSE, FALSE, FALSE, FALSE, FALSE, FALSE, FALSE, FALSE, FALSE, FALSE], "Connection Type"=enum."Disconnected"}, {"Connections"=[FALSE, FALSE, FALSE, FALSE, FALSE, FALSE, FALSE, FALSE, FALSE, FALSE, FALSE, FALSE], "Connection Type"=enum."Disconnected"}, {"Connections"=[FALSE, FALSE, FALSE, FALSE, FALSE, FALSE, FALSE, FALSE, FALSE, FALSE, FALSE, FALSE], "Connection Type"=enum."Disconnected"}, {"Connections"=[FALSE, FALSE, FALSE, FALSE, FALSE, FALSE, FALSE, FALSE, FALSE, FALSE, FALSE, FALSE], "Connection Type"=enum."Disconnected"}]}, "Refnums"={"Connections"=refnum, "Instrument Status"=refnum}, "Initialization"={"Update Visa Session"=FALSE, "Update Refnums"=FALSE}}, "Stress Control"={"Configuration"={"Stress Control VISA Session"="StrainMotor", "Axis"=0, "Motion"=0, "Destination (°)"=0.0, "Speed (°/s)"=4.0, "Position (°)"=25.0}, "Refnums"={"Instrument Status"=refnum, "Position"=refnum, "Mecahnism Motion"=refnum, "Destination"=refnum, "Apply Stress"=refnum, "Stop"=refnum, "Stress Control VISA"=refnum}, "Initialization"={"Update Visa Session"=FALSE, "Update Configuration"=FALSE, "Update Refnums"=FALSE, "Get Position"=FALSE}}, "Optical Spectrometer"={"Configuration"={"Laser Settings"={"Laser Wavelength"=enum."784 nm", "Neutral Density Filter"=enum."50%"}, "Spectrometer Settings"={"Confocal Hole Size (µm)"=150.0, "Grating"=2, "Detector"=enum."InGaAs Array"}, "Acquisition Settings"={"Acquisition Mode"=enum."Multi-Window", "Spectal Position (nm)"=632.0, "From (nm)"=735.0, "To (nm)"=3.0, "Integration Time (s)"=3.0, "Number of Accumulations"=3, "AutoScanning"=FALSE, "Spike Removal"=FALSE}, "Path"=path "C:/07 - Prizes and Awards/Marie Curie Prize/Reply Editors Final NCOMMS(10).docx"}, "Refnums"={"Instrument Status"=refnum, "Optical Spectrum Plot"={"Plot List"=refnum, "Optical Spectrum vs Energy"=refnum, "Optical Spectrum vs Wavelength"=refnum, "Optical Spectrum vs Raman Shift"=refnum, "Detector Temperature"=refnum}, "Laser"=refnum, "Filter"=refnum, "Laser ON?"=refnum, "Hole"=refnum, "Grating"=refnum, "Detector"=refnum, "Acquisition Mode"=refnum, "Spectal Position"=refnum, "From"=refnum, "To"=refnum, "Integration Time"=refnum, "Accumulations"=refnum, "AutoScanning"=refnum, "Spike Removal"=refnum, "Acquisition Mode Panel"=refnum}, "Initialization"={"Connect"=FALSE, "Update Refnums"=FALSE, "Get Configuration"=FALSE}}, "Switches & Mirrors"={"Configuration"={"Relay VISA Session"="COM1", "Switches"={"Laser"=FALSE, "Video"=FALSE}, "Delays (ms)"={"Laser"=500, "Video"=1500}}, "Refnums"={"Instrument Status"=refnum, "Laser"=refnum, "Video"=refnum, "Relay VISA"=refnum}, "Initialize"={"Update Refnums"=FALSE, "Connect"=FALSE, "Set Configuration"=FALSE}}, "Camera"={"Configuration"={"Settings"={"Pixel clock"=20, "Frame rate"=30.0, "Exposure time"=33.21525, "Master Gain"=0, "Red Gain"=0, "Green Gain"=0, "Blue Gain"=0, "Auto Gain"=FALSE, "White-balance"=FALSE, "Color Correction"=FALSE}}, "Refnums"={"Pixel Clock"=refnum, "Frame Rate"=refnum, "Exposure Time"=refnum, "Master Gain"=refnum, "Red Gain"=refnum, "Green Gain"=refnum, "Blue Gain"=refnum, "Auto Gain"=refnum, "Auto White-balance"=refnum, "Color Correction"=refnum, "Image"=refnum, "Video Button"=refnum, "Instrument Status"=refnum}, "Initialization"={"Connect"=FALSE, "Update Refnums"=FALSE, "Acquiring?"=FALSE}}, "XYZ Stage"={"Configuration"={"Connection Settings"={"Tango VISA"="", "Baudrate"=57600, "Show Protocol?"=FALSE}, "Manual Control"={"North"=FALSE, "South"=FALSE, "West"=FALSE, "East"=FALSE, "Up"=FALSE, "Down"=FALSE, "Stop"=FALSE, "XY Step"=0.0, "Z step"=0.0}, "Coordinate Control"={"Motion Mode"=enum."Absolute", "Destination [mm]"=[]}}, "Refnums"={"Instrument Status"=refnum, "Position"=refnum, "Manual Control"=refnum, "Up"=refnum, "Down"=refnum, "North"=refnum, "South"=refnum, "East"=refnum, "West"=refnum, "Stop"=refnum, "Limits"=refnum}, "Initialization"={"Update Visa Session"=FALSE, "Set To Default"=FALSE, "Get Status"=FALSE, "Update Refnums"=FALSE}}, "AutoFocus"={"Configuration"={"Matching Criteria"={"Minimum Score"=700.0, "Color Score Weight"=700.0, "Minimum Contrast"=50, "Match Mode"=0, "Match Feature Mode"=0, "Subpixel Accuracy"=TRUE, "Color Sensitivity"=1, "Search Strategy"=1}, "Z Scan Parameters"={"Z Range"=1380.0, "Resolution"=5000.0, "Initial Direction"=enum."Up", "Focus Threshold"=0.1, "Ascent Constant"=0.1}, "Displacement"=0.0, "Transformation Matrix"=[]}, "Refnums"={"Instrument Status"=refnum, "Matching Criteria"=refnum, "Z Scan Parameters"=refnum, "Distance"=refnum, "Transformation Matrix"=refnum, "Match and Edge"={"Image"=refnum, "Target"=refnum, "Edge"=refnum, "Target Data"=refnum}, "Matching Curves"=refnum, "Tracking"=refnum, "Focus"=refnum, "Find Focus"=refnum, "Set Target"=refnum, "Link Stage & Camera"=refnum, "Align"=refnum}, "Initialize"={"Update Refnums"=FALSE, "Allocate Image Memory"=FALSE, "Set Match Criteria"=FALSE, "Link Stage & Camera"=FALSE, "Set Target"=FALSE, "Find Target"=FALSE}}} ("Instruments Status")
        n5 = Unbundle By Name(w32) -> ("Parameter Analyzer.Instrument Data"=w37:refnum<notifier>, "Optical Spectrometer.Instrument Data"=w24:refnum<notifier>)
        n6 = Cancel Notification(0:w24, 3:w35) -> (11:w44:errorcluster)  [unwired: 2 out]
        n7 = Cancel Notification(0:w37, 3:w35) -> (11:w42:errorcluster)  [unwired: 2 out]
        n8 = Merge Errors(w42, w44) -> (w27:errorcluster)
        n9 = Unbundle By Name(w33) -> ("Optical Spectrometer"=w47:refnum<queue>, "Parameter Analyzer"=w48:refnum<queue>)
        n10 = Unbundle By Name(w50) -> ("Parameter Analyzer"=w36:T39, "Optical Spectrometer"=w38:T56)
        n11 = Wait on Notification(notifier=w37, error in (no error)=w27) -> (notification=w39:variant, error out=w40:errorcluster)  [unwired: 4 out]
        n12 = Wait on Notification(notifier=w24, error in (no error)=w27) -> (notification=w28:variant, error out=w29:errorcluster)  [unwired: 4 out]
        n13 = call "Enqueue Message (Single).vi"("error in (no error)"=w27, "Message"=w49, "Message Queue"=w47) -> ("error out"=w26:errorcluster)  [unwired: 1 in, 7 out]
        n14 = call "Enqueue Message (Single).vi"("error in (no error)"=w27, "Message"=w49, "Message Queue"=w48) -> ("error out"=w25:errorcluster)  [unwired: 1 in, 7 out]
        n15 = Variant To Data(error in=w29, type=w38, Variant=w28) -> (data=w46:T56, error out=w45:errorcluster)
        n16 = Variant To Data(error in=w40, type=w36, Variant=w39) -> (data=w41:T39, error out=w43:errorcluster)
        n17 = Bundle By Name(cluster=w50, "Parameter Analyzer"=w41, "Optical Spectrometer"=w46) -> (w34:T38)
        n18 = Merge Errors(w43, w45, w26, w25) -> (w30:errorcluster)
      }
      frame "Measure" {
        w87 = "Measurement Performed"  # Status
        # "Data Saved in \nWorkspace by \nTool already"
        n19 = Unbundle By Name(w55) -> ("Parameter Analyzer.Measurement"=w104:refnum<notifier>, "Optical Spectrometer.Measurement"=w105:refnum<notifier>)
        n20 = Unbundle By Name(w70) -> ("Instrument Status"=w75:refnum<vi>)
        n21 = control-ref of="Instrument Status"() -> (w76:refnum<vi>)
        n22 = Unbundle By Name(w61) -> ("Parameter Analyzer.Configuration.Acquisition Mode"=w51:enum32{"Sweeping Mode", "Sampling Mode"})
        n23 = Unbundle By Name(w61) -> ("Parameter Analyzer.Configuration"=w96:T40)
        n24 = call "Edit All Status Indicators.vi"("Instrument Status Ouside"=w75, "Instrument Status Inside"=w76, "Error In"=w74, "State"=Instrument_Status_State."Measuring") -> ("Error Out"=w73:errorcluster)  [unwired: 6 in]
        n25 = Cancel Notification(0:w105, 3:w73) -> (8:w106:refnum<notifier>, 11:w113:errorcluster)  [unwired: 1 out]
        n26 = Cancel Notification(0:w104, 3:w73) -> (8:w99:refnum<notifier>, 11:w103:errorcluster)  [unwired: 1 out]
        n27 = Unbundle By Name(w60) -> ("Parameter Analyzer"=w97:refnum<queue>)
        n28 = Merge Errors(w103, w113) -> (w95:errorcluster)
        n29 = case shown="\"Sampling Mode\"" w51 {
          tunnel: [enum16{"Sweeping Mode", "Sampling Mode"}."Sweeping Mode" ("Measurement Mode") enum16{"Sweeping Mode", "Sampling Mode"}."Sampling Mode" ("Measurement Mode")] -> w52
          frame "Sweeping Mode", Default {
          }
          frame "Sampling Mode" {
          }
        }
        n30 = Wait on Notification(notifier=w99, error in (no error)=w95) -> (notification=w101:variant, error out=w100:errorcluster)  [unwired: 4 out]
        n31 = Wait on Notification(notifier=w106, error in (no error)=w95) -> (notification=w108:variant, error out=w109:errorcluster)  [unwired: 4 out]
        n32 = Variant To Data(error in=w100, type=T36 {"Sequence"=[], "V1"=[], "V2"=[], "V3"=[], "V4"=[], "I1"=[], "I2"=[], "I3"=[], "I4"=[]} ("Measurement"), Variant=w101) -> (data=w68:T36, error out=w94:errorcluster)
        n33 = Variant To Data(error in=w109, type=T35 {"Intensity"=[], "Wavelength"=[], "Energy"=[], "Raman Shift"=[], "Detector Temperature"=0.0} ("Measurement"), Variant=w108) -> (data=w67:T35, error out=w91:errorcluster)
        n34 = call "Enqueue Message (Single).vi"("error in (no error)"=w95, "Message Data"=w96, "Message"="Measure", "Message Queue"=w97) -> ("error out"=w58:errorcluster)  [unwired: 7 out]
        n35 = Unbundle By Name(w55) -> ("Parameter Analyzer.Status"=w56:refnum<notifier>)
        n36 = Unbundle By Name(w70) -> ("Electrical Data Plot"=w72:T3)
        n37 = Unbundle By Name(w70) -> ("Optical Spectrum Plot"=w71:T2)
        n38 = call "Wait for event.vi"("error in (no error)"=w58, "String"="Measuring", "Notifier in"=w56) -> ("error out"=w57:errorcluster)  [unwired: 7 in, 1 out]
        n39 = call "Plot Electrical Data.vi"("Plot Refnums"=w72, "Plot List"=T33."Current & Voltage Traces", "Electrical Measurement"=w68, "Measurement Mode"=w52, "error in (no error)"=w94, "Update Labels?"=TRUE) -> ("Voltage Plot Array"=→"Voltage Plot":cluster{"Sequence":dbl[], "Data":dbl[]}[], "Current Plot Array"=→"Current Plot":cluster{"Sequence":dbl[], "Data":dbl[]}[], "error out"=w89:errorcluster)  [unwired: 1 in, 6 out]
        n40 = Unbundle By Name(w60) -> ("Optical Spectrometer"=w111:refnum<queue>)
        n41 = call "Plot Spectrum.vi"("Optical Spectrum Plot"=w71, "Spectrum"=w67, "error in (no error)"=w91) -> ("Optical Spectrum vs Energy"=→"Optical Spectrum vs Energy":cluster{"data":dbl[], "data":dbl[]}, "Optical Spectrum vs Wavelength"=→"Optical Spectrum vs Wavelength":cluster{"data":dbl[], "data":dbl[]}, "Optical Spectrum vs Raman Shift"=→"Optical Spectrum vs Raman Shift":cluster{"data":dbl[], "data":dbl[]}, "error out"=w90:errorcluster)  [unwired: 9 in]
        n42 = Bundle By Name(cluster=T34 {"Optical Spectrum"={"Intensity"=[], "Wavelength"=[], "Energy"=[], "Raman Shift"=[], "Detector Temperature"=0.0}, "Electrical Measurement"={"Sequence"=[], "V1"=[], "V2"=[], "V3"=[], "V4"=[], "I1"=[], "I2"=[], "I3"=[], "I4"=[]}} ("Measurement"), "Electrical Measurement"=w68, "Optical Spectrum"=w67) -> (w62:T34)
        n43 = call "Enqueue Message (Single).vi"("error in (no error)"=w57, "Message"="Acquire Spectrum", "Message Queue"=w111) -> ("error out"=w112:errorcluster)  [unwired: 1 in, 7 out]
        n44 = Unbundle By Name(w55) -> ("Optoelectronic.Status"=w86:refnum<notifier>, "Optoelectronic.Measurement"=w64:refnum<notifier>)
        n45 = Merge Errors(w112, w89, w90) -> (w65:errorcluster)
        n46 = Unbundle By Name(w70) -> ("Instrument Status"=w81:refnum<vi>)
        n47 = control-ref of="Instrument Status"() -> (w80:refnum<vi>)
        n48 = Not A Number/Path/Refnum?(number/path/refnum=w64) -> (NaN/Path/Refnum?=w66:bool)
        n49 = case shown="False" w66 {
          tunnel: w65 -> [w119 w120]
          tunnel: [w118 w120] -> w63
          tunnel: w64 -> [w117 _]
          tunnel: w62 -> [w116 _]
          frame False {
            n50 = Send Notification(notification=w116, notifier=w117, error in (no error)=w119) -> (error out=w118:errorcluster)  [unwired: 1 out]
          }
          frame True {
          }
        }
        n51 = call "Edit All Status Indicators.vi"("Instrument Status Ouside"=w81, "Instrument Status Inside"=w80, "Error In"=w65, "State"=Instrument_Status_State."Idle") -> ("Error Out"=w78:errorcluster)  [unwired: 6 in]
        n52 = call "Notify.vi"("error in (no error)"=w63, "String"=w87, "Notifier in"=w86) -> ("error out"=w88:errorcluster)  [unwired: 8 in]
        n53 = Merge Errors(w88, w78) -> (w85:errorcluster)
      }
      frame "Set Parameter Analyzer", Default {
      }
      frame "Set Spectrometer" {
      }
      frame "Set Acquisition" {
      }
    }
  }
  "error out" <- w1
